vi "HART_Unpack ASCII.vi"(11 "Read Packed ASCII String":string) -> (3 "Array":u8[](array[numeric]) format="%.0x")   [LabVIEW 2010]
doc: "Reconstruction of ASCII characters from Packed (6bist ASCII) data format"
panel:
  out "UNPACKED 2d 8 bits array ALL":bool[][](array[boolean])
  out "Rest 8Bits Array":bool[][](array[boolean])
  out "UNPACKED 2d 8 bits array":bool[][](array[boolean])
  out "Numeric":i32
  out "size(s)":i32
  out "2d 24 bits array":bool[][](array[boolean])
  out "All bits in one array":bool[](array[boolean])
  out "2d 8bits array":bool[][](array[boolean])
  out "hex integer string 2":string[](array[string])
  out "unsigned byte array":u8[](array[numeric]) format="%.0b"
  out "length":i32
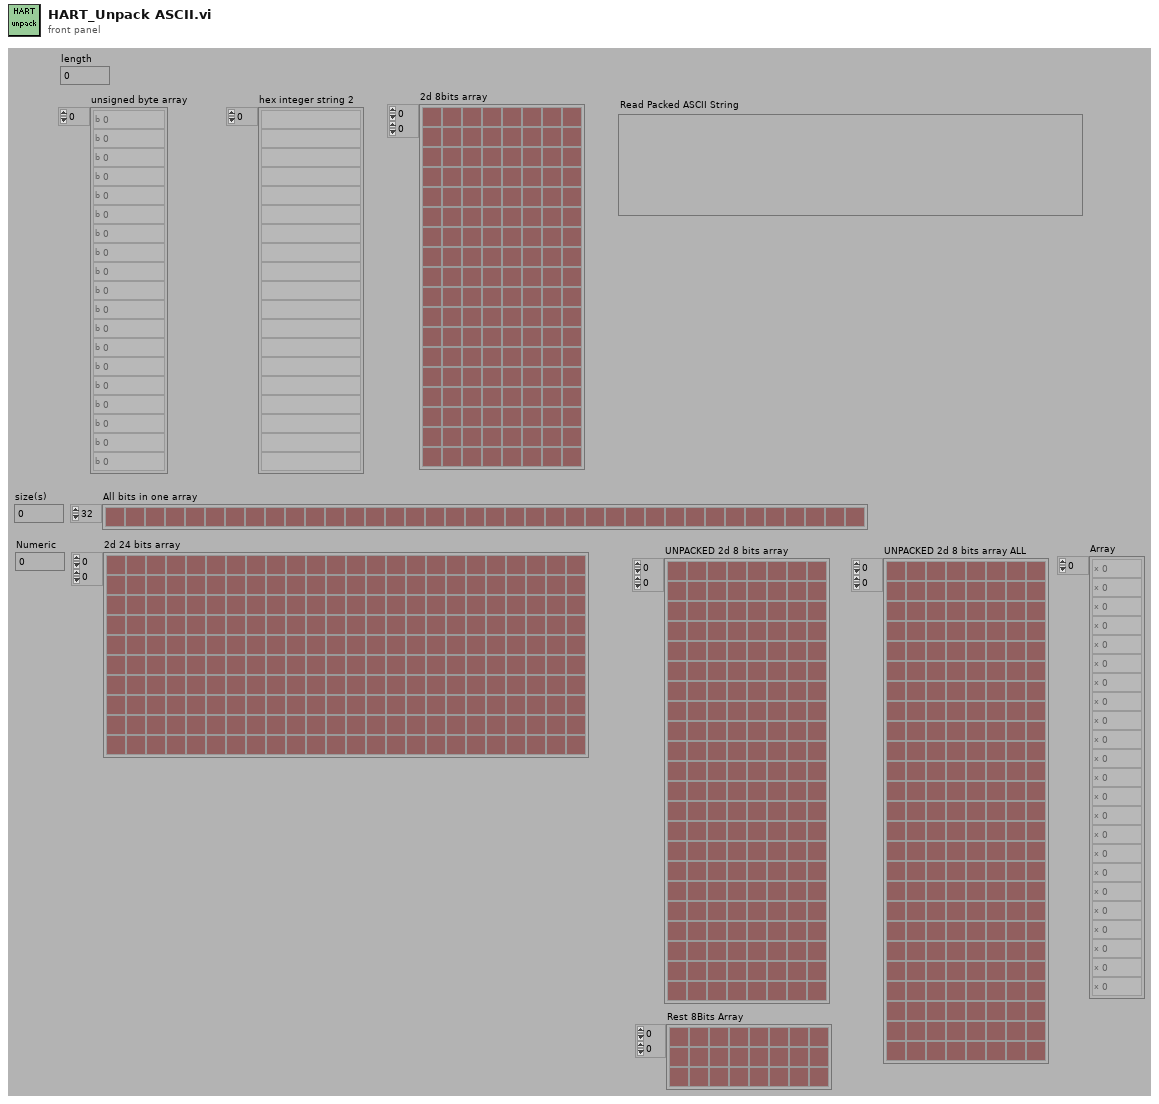
[diagram p1: front panel]
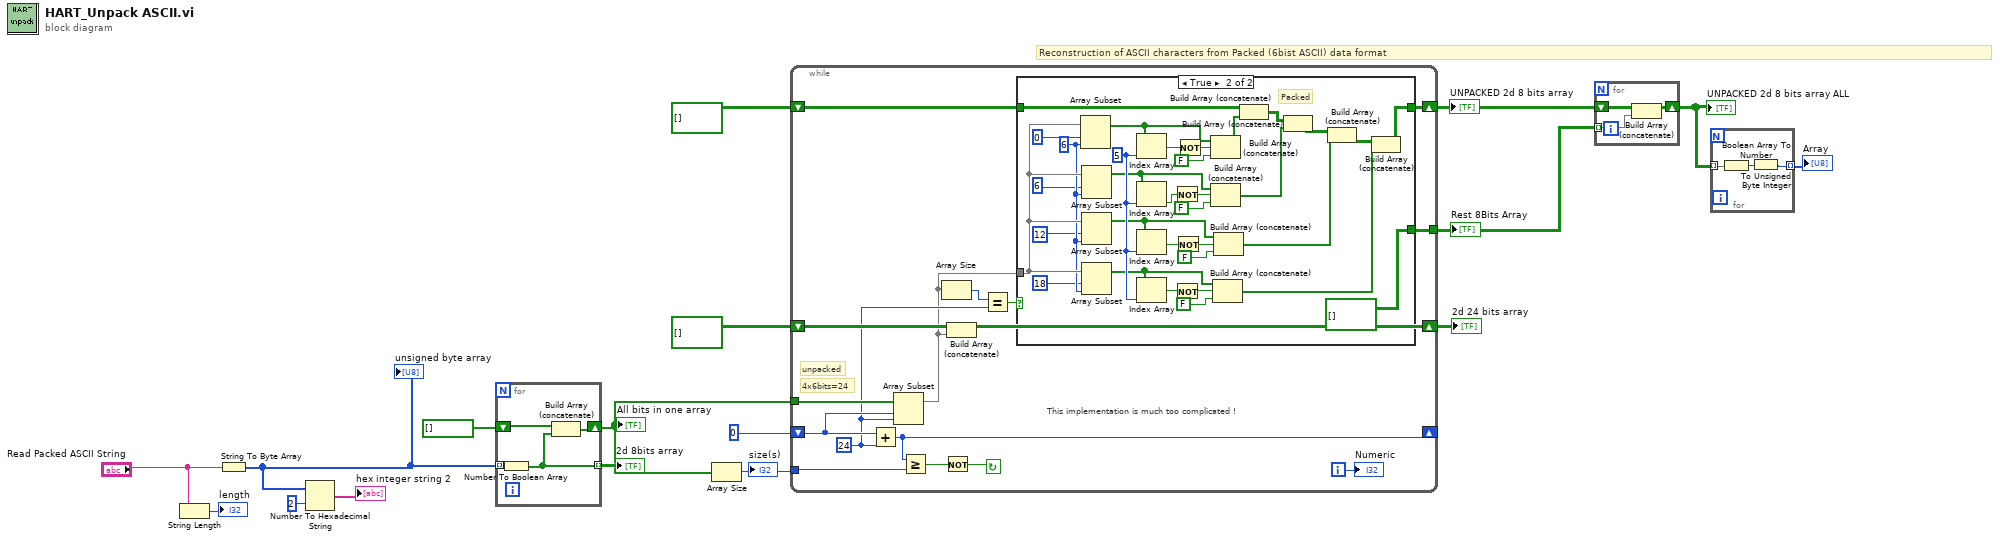
[diagram p0: block diagram]
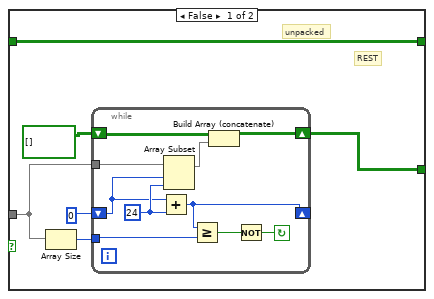
[diagram p2: hidden frame]
diagram:
  # "Reconstruction of ASCII characters from Packed (6bist ASCII) data format"
  n1 = String Length(string="Read Packed ASCII String") -> (length=→"length":i32)
  n2 = String To Byte Array(string="Read Packed ASCII String") -> (unsigned byte array=w15:u8[])
  "unsigned byte array" <- w15
  n3 = Number To Hexadecimal String(1:i16 2 ("width (-)"), 2:w15) -> (0:→"hex integer string 2":string[])
  n4 = for {
    tunnel: w15 -> [w21] mode=indexing
    tunnel: [w20] -> w12 mode=indexing
    shift-right: [w18] -> w9
    shift-left: bool[] [] ("Boolean array 2") -> [w19]
    n5 = Number To Boolean Array(number=w21) -> (Boolean array=w20:bool[])
    n6 = Build Array (concatenate)(w19, w20) -> (w18:bool[])
  }
  "2d 8bits array" <- w12
  "All bits in one array" <- w9
  n7 = Array Size(array=w9) -> (size(s)=w8:i32)
  "size(s)" <- w8
  n8 = while {
    tunnel: [w22] -> w3
    shift-left: bool[][] [] ("2d Boolean array") -> [w28]
    shift-right: [w27] -> w4
    shift-left: bool[][] [] ("2d Boolean array") -> [w32]
    shift-right: [w31] -> w6
    tunnel: w8 -> [w34]
    tunnel: w9 -> [w36]
    shift-left: i16 0 ("width (-)") -> [w37]
    shift-right: [w35] -> _
    i -> [w30]
    stop <- w29 continue-if-true
    w25 = 24 ("length")
    # "This implementation is much too complicated !"
    # "unpacked"
    # "4x6bits=24"
    n9 = Add(x=w37, y=w25) -> (x+y=w35:i32)
    n10 = Array Subset(array=w36, index=w37, length=w25) -> (w23:bool[])
    n11 = Greater Or Equal?(x=w35, y=w34) -> (x >= y?=w33:bool)
    n12 = Array Size(array=w23) -> (size(s)=w26:i32)
    n13 = Not(x=w33) -> (.not. x?=w29:bool)
    n14 = Build Array (concatenate)(w32, w23) -> (w31:bool[][])
    n15 = Equal?(x=w26, y=w25) -> (x = y?=w24:bool)
    n16 = case shown="True" w24 {
      tunnel: w28 -> [w43 w85]
      tunnel: [w43 w82] -> w27
      tunnel: w23 -> [w42 w81]
      tunnel: [w38 bool[][] [] ("2d Boolean array")] -> w22
      frame False {
        # "REST"
        # "unpacked"
        n17 = Array Size(array=w42) -> (size(s)=w41:i32)
        n18 = while {
          shift-left: bool[][] [] ("2d Boolean array") -> [w46]
          shift-right: [w44] -> w38
          shift-left: i16 0 ("width (-)") -> [w51]
          shift-right: [w48] -> _
          tunnel: w41 -> [w50]
          tunnel: w42 -> [w49]
          stop <- w47 continue-if-true
          w53 = 24 ("length")
          n19 = Add(x=w51, y=w53) -> (x+y=w48:i32)
          n20 = Array Subset(array=w49, index=w51, length=w53) -> (w45:bool[])
          n21 = Greater Or Equal?(x=w48, y=w50) -> (x >= y?=w52:bool)
          n22 = Build Array (concatenate)(w46, w45) -> (w44:bool[][])
          n23 = Not(x=w52) -> (.not. x?=w47:bool)
        }
      }
      frame True {
        w75 = 5 ("Index")
        w80 = 6 ("Array Length")
        # "Packed"
        n24 = Array Subset(array=w81, index=0 ("Array Index"), length=w80) -> (w73:bool[])
        n25 = Array Subset(array=w81, index=6 ("Array Index"), length=w80) -> (w66:bool[])
        n26 = Array Subset(array=w81, index=12 ("Array Index"), length=w80) -> (w67:bool[])
        n27 = Array Subset(array=w81, index=18 ("Array Index"), length=w80) -> (w68:bool[])
        n28 = Index Array(array=w73, index=w75) -> (element=w74:bool)
        n29 = Index Array(array=w66, index=w75) -> (element=w65:bool)
        n30 = Index Array(array=w67, index=w75) -> (element=w64:bool)
        n31 = Index Array(array=w68, index=w75) -> (element=w63:bool)
        n32 = Not(x=w65) -> (.not. x?=w56:bool)
        n33 = Not(x=w63) -> (.not. x?=w54:bool)
        n34 = Not(x=w64) -> (.not. x?=w55:bool)
        n35 = Not(x=w74) -> (.not. x?=w57:bool)
        n36 = Build Array (concatenate)(w73, w57, FALSE ("Input Element")) -> (w62:bool[])
        n37 = Build Array (concatenate)(w66, w56, FALSE ("Input Element")) -> (w61:bool[])
        n38 = Build Array (concatenate)(w68, w54, FALSE ("Input Element")) -> (w59:bool[])
        n39 = Build Array (concatenate)(w67, w55, FALSE ("Input Element")) -> (w60:bool[])
        n40 = Build Array (concatenate)(w85, w62) -> (w86:bool[][])
        n41 = Build Array (concatenate)(w86, w61) -> (w84:bool[][])
        n42 = Build Array (concatenate)(w84, w60) -> (w83:bool[][])
        n43 = Build Array (concatenate)(w83, w59) -> (w82:bool[][])
      }
    }
    "Numeric" <- w30
  }
  "2d 24 bits array" <- w6
  "UNPACKED 2d 8 bits array" <- w4
  "Rest 8Bits Array" <- w3
  n44 = for {
    tunnel: w3 -> [w89] mode=indexing
    shift-right: [w87] -> w2
    shift-left: w4 -> [w88]
    n45 = Build Array (concatenate)(w88, w89) -> (w87:bool[][])
  }
  "UNPACKED 2d 8 bits array ALL" <- w2
  n46 = for {
    tunnel: w2 -> [w92] mode=indexing
    tunnel: [w90] -> w1 mode=indexing
    n47 = Boolean Array To Number(Boolean array=w92) -> (number=w91:u32)
    n48 = To Unsigned Byte Integer(number=w91) -> (unsigned 8bit integer=w90:u8)
  }
  "Array" <- w1
